vi "Math-Rectangles Intersect.vi"(5 "Rect1":T1, 9 "Rect2":T1) -> (8 "intersect?":bool)   [LabVIEW 2015]
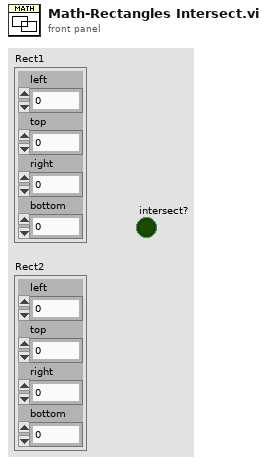
[diagram p1: front panel]
types:
  T1 = cluster{"left":i16, "top":i16, "right":i16, "bottom":i16}
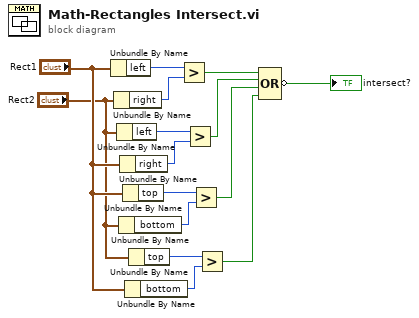
[diagram p0: block diagram]
diagram:
  n1 = Unbundle By Name("Rect1") -> ("left"=w15:i16)
  n2 = Unbundle By Name("Rect2") -> ("right"=w14:i16)
  n3 = Unbundle By Name("Rect2") -> ("left"=w13:i16)
  n4 = Unbundle By Name("Rect2") -> ("bottom"=w9:i16)
  n5 = Unbundle By Name("Rect1") -> ("right"=w12:i16)
  n6 = Unbundle By Name("Rect1") -> ("top"=w11:i16)
  n7 = Unbundle By Name("Rect1") -> ("bottom"=w8:i16)
  n8 = Unbundle By Name("Rect2") -> ("top"=w10:i16)
  n9 = Greater?(x=w15, y=w14) -> (0:w5:bool)
  n10 = Greater?(x=w13, y=w12) -> (0:w4:bool)
  n11 = Greater?(x=w11, y=w9) -> (0:w3:bool)
  n12 = Greater?(x=w10, y=w8) -> (0:w2:bool)
  n13 = Compound Arithmetic op=OR(w5, w4, w3, w2) -> (invert →"intersect?":bool)
